vi "Zadanie_2.vi"() -> ()   [LabVIEW 2024]
panel:
  in  "stop":bool
  out "Liczba \nAktywnych":i16
  in  "4":bool
  in  "3":bool
  in  "2":bool
  in  "1":bool
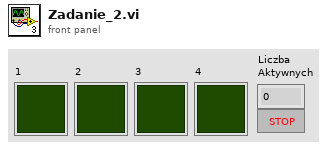
[diagram p1: front panel]
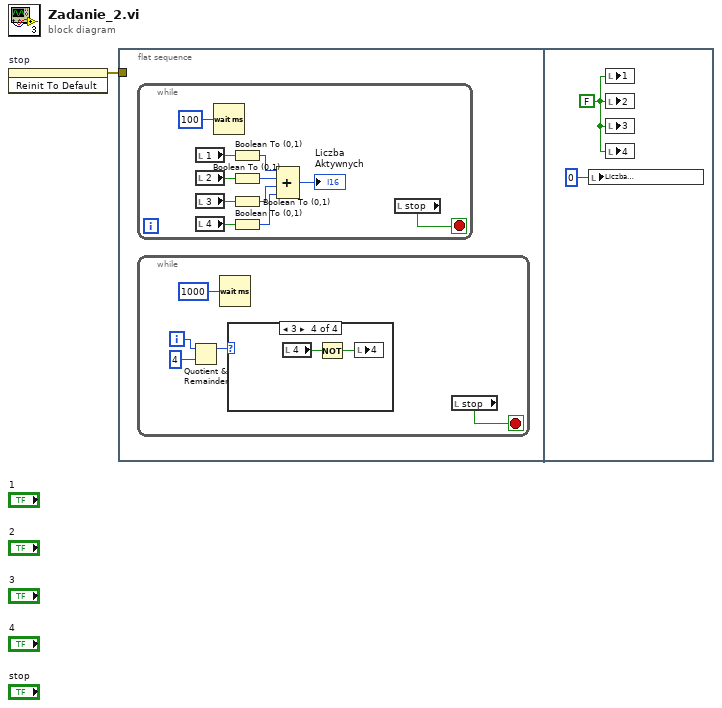
[diagram p0: block diagram]
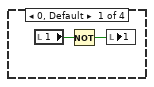
[diagram p2: hidden frame]
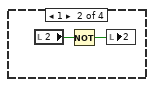
[diagram p3: hidden frame]
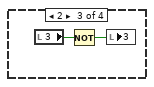
[diagram p4: hidden frame]
diagram:
  n1 = invoke on="stop" class="Bool (strict)" method="Reinit To Default"() -> (error out=w1:errorcluster)  [unwired: 3 in, 2 out]
  n2 = flat-sequence {
    tunnel: w1 -> [_]
    frame #0 {
      n3 = while {
        stop <- w2 stop-if-true
        n4 = local read "1"() -> (w11:bool)
        n5 = local read "2"() -> (w9:bool)
        n6 = local read "3"() -> (w8:bool)
        n7 = local read "4"() -> (w7:bool)
        n8 = Wait (ms)(milliseconds to wait=u32 100) -> ()  [unwired: 1 out]
        n9 = Boolean To (0,1)(Boolean=w11) -> (0, 1=w10:i16)
        n10 = Boolean To (0,1)(Boolean=w9) -> (0, 1=w6:i16)
        n11 = Boolean To (0,1)(Boolean=w8) -> (0, 1=w5:i16)
        n12 = Boolean To (0,1)(Boolean=w7) -> (0, 1=w4:i16)
        n13 = Compound Arithmetic op=ADD(w10, w6, w5, w4) -> (→"Liczba \nAktywnych":i16)
        n14 = local read "stop"() -> (w2:bool)
      }
      n15 = while {
        i -> [w15]
        stop <- w13 stop-if-true
        n16 = Quotient & Remainder(x=w15, y=4) -> (x-y*floor(x/y)=w14:i32)  [unwired: 1 out]
        n17 = Wait (ms)(milliseconds to wait=u32 1000) -> ()  [unwired: 1 out]
        n18 = case shown="3" w14 {
          frame 0, Default {
            n19 = local read "1"() -> (w19:bool)
            n20 = Not(x=w19) -> (.not. x?=w18:bool)
            n21 = local write "1"(w18) -> ()
          }
          frame 1 {
            n22 = local read "2"() -> (w21:bool)
            n23 = Not(x=w21) -> (.not. x?=w20:bool)
            n24 = local write "2"(w20) -> ()
          }
          frame 2 {
            n25 = local read "3"() -> (w23:bool)
            n26 = Not(x=w23) -> (.not. x?=w22:bool)
            n27 = local write "3"(w22) -> ()
          }
          frame 3 {
            n28 = local read "4"() -> (w25:bool)
            n29 = Not(x=w25) -> (.not. x?=w24:bool)
            n30 = local write "4"(w24) -> ()
          }
        }
        n31 = local read "stop"() -> (w13:bool)
      }
    }
    frame #1 {
      w26 = FALSE ("4")
      n32 = local write "Liczba \nAktywnych"(i16 0 ("Liczba \nAktywnych")) -> ()
      n33 = local write "1"(w26) -> ()
      n34 = local write "2"(w26) -> ()
      n35 = local write "3"(w26) -> ()
      n36 = local write "4"(w26) -> ()
    }
  }
